vi "Loop.vi"(11 "Base Server in":refnum<class "Server.lvclass">) -> ()   [LabVIEW 2024, in "Ramses Framework.lvlib" / "Server.lvclass"]
uses:
  Server.lvclass
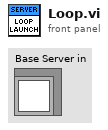
[diagram p1: front panel]
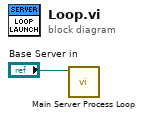
[diagram p0: block diagram]
diagram:
  n1 = call-dynamic "Main Server Process Loop.vi"("Base Server in"="Base Server in") -> ()  [unwired: 11 in]
